vi "Untitled 1.vi"() -> ()   [LabVIEW 2020]
uses:
  <vilib>/Analysis/polynomials.llb/Polynomial Roots (DBL).vi
  <vilib>/Analysis/NI_AALPro.lvlib
panel:
  out "Roots":cdb[](array[numeric])
  out "x2":dbl
  out "x1":dbl
  in  "c":dbl
  in  "b":dbl
  in  "a":dbl
  # "(3x^2)+3x+4"
  # "Ahmed Göktuğ Aydın - 200208054"
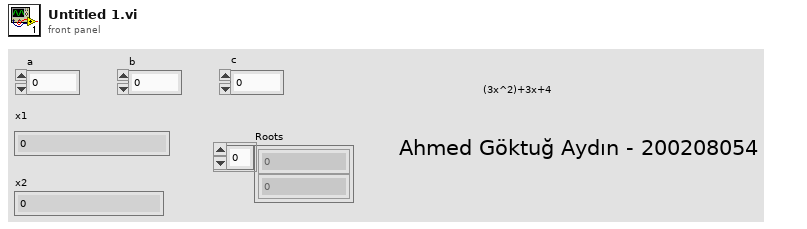
[diagram p1: front panel]
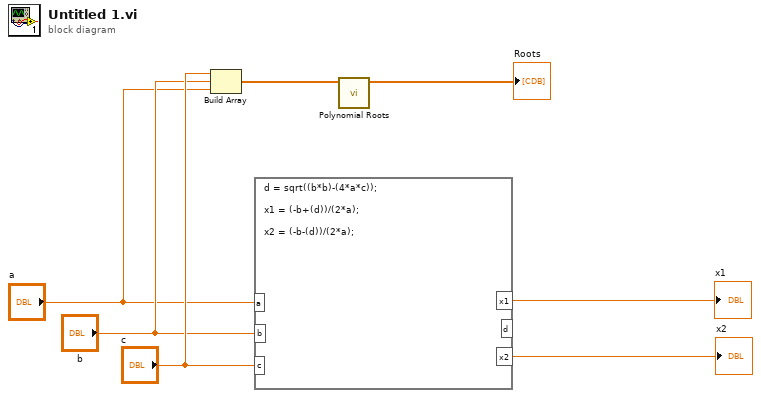
[diagram p0: block diagram]
diagram:
  n1 = Build Array("c", "b", "a") -> (w4:dbl[])
  n2 = formula code="d = sqrt((b*b)-(4*a*c));\n\nx1 = (-b+(d))/(2*a);\n\nx2 = (-b-(d))/(2*a);"("a"="a", "b"="b", "c"="c") -> ("x1"=→"x1":dbl, "x2"=→"x2":dbl)  [unwired: 1 out]
  n3 = call-poly <vilib>:"Polynomial Roots.vi"("P(x)"=w4) -> ("Roots"=→"Roots":cdb[])  [unwired: 9 in, 1 out]
